vi "Trainging_OneClick.vi"() -> ()   [LabVIEW 2014]
uses:
  <vilib>/Utility/file.llb/Read From Spreadsheet File (string).vi
  <vilib>/Utility/file.llb/Read From Spreadsheet File (I64).vi
  <vilib>/Utility/file.llb/Read From Spreadsheet File (DBL).vi
  <vilib>/Utility/file.llb/Write To Spreadsheet File (DBL).vi
  <vilib>/Utility/file.llb/Write To Spreadsheet File (I64).vi
panel:
  out "error out 2":errorcluster
  out "error out":errorcluster
  out "Path_error out":errorcluster
  in  "Training_Path":path
  in  "Random_num":i32=6
  in  "Flash_Repeat":i32=20
  in  "Frame_Length":i32=20
  in  "Variables":T1={"s_verbose"=enum."On", "displayInterval"=1.0, "displayMode"=enum."On", "sampleSize"=1.0, "guess"=[[1.0]], "initState"=enum."rand", "maxFinetune"=100.0, "maxNumIteration"=100.0, "epsilon"=0.0001, "stabilization"=enum."On", "myy"=1.0, "a1"=1.0, "a2"=1.0, "finetune"=enum."off", "g"=enum."pow3", "approach"=enum."symm"}
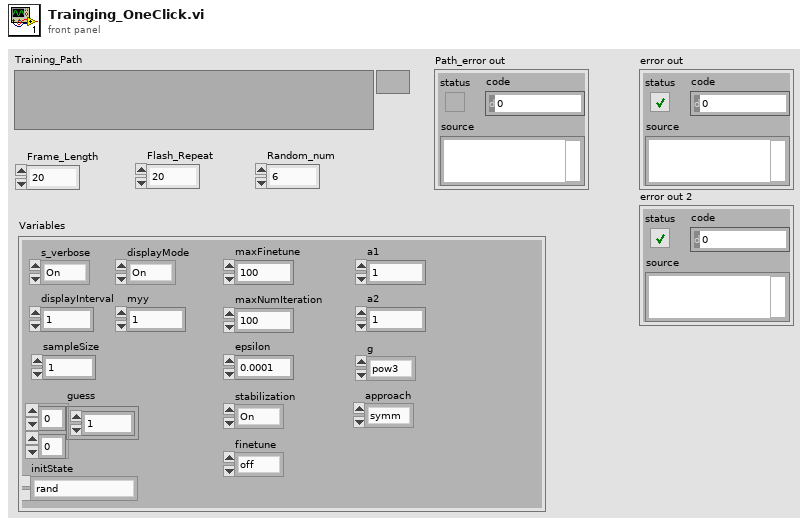
[diagram p1: front panel]
types:
  T1 = cluster{"s_verbose":enum16{"Off", "On"}, "displayInterval":dbl, "displayMode":enum16{"Off", "On"}, "sampleSize":dbl, "guess":dbl[][], "initState":enum16{"rand", "guess"}, "maxFinetune":dbl, "maxNumIteration":dbl, "epsilon":dbl, "stabilization":enum16{"Off", "On"}, "myy":dbl, "a1":dbl, "a2":dbl, "finetune":enum16{"pow3", "tanh", "gauss", "skew", "off"}, "g":enum16{"pow3", "tanh", "gauss", "skew"}, "approach":enum16{"symm", "delf"}}
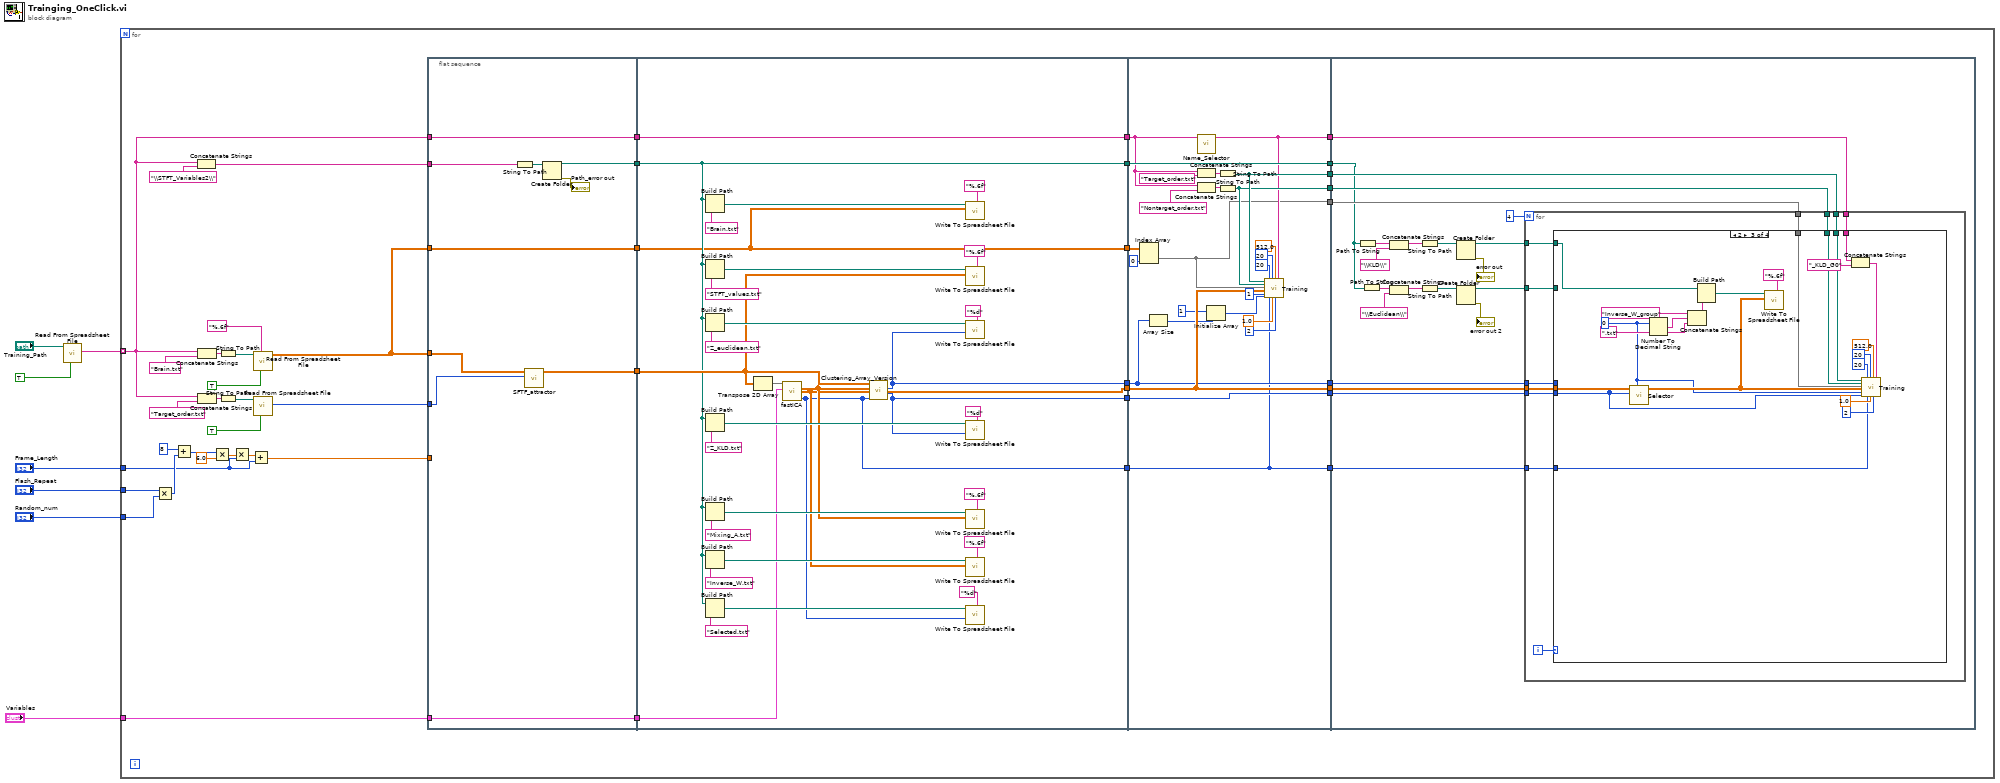
[diagram p0: block diagram]
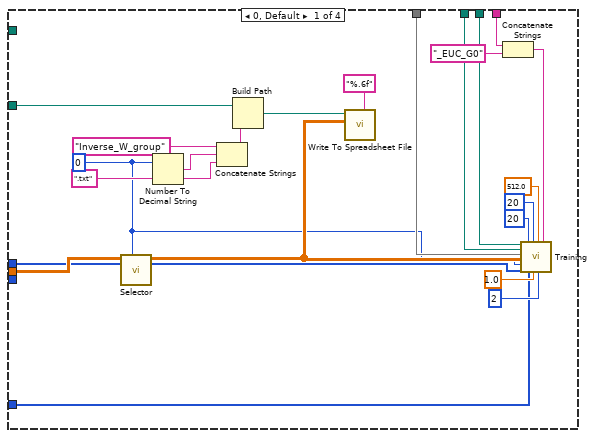
[diagram p2: hidden frame]
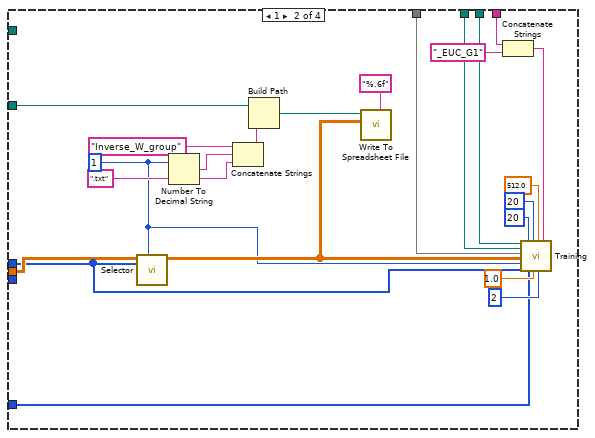
[diagram p3: hidden frame]
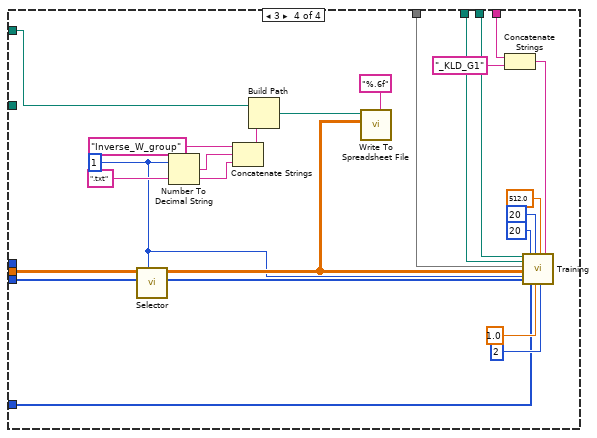
[diagram p4: hidden frame]
diagram:
  n1 = call-poly <vilib>:"Read From Spreadsheet File.vi"("transpose (no:F)"=TRUE, "file path (dialog if empty)"="Training_Path") -> ("first row"=w5:string[])  [unwired: 5 in, 4 out]
  n2 = for {
    tunnel: w5 -> [w9] mode=indexing
    tunnel: "Frame_Length" -> [w39]
    tunnel: "Flash_Repeat" -> [w38]
    tunnel: "Random_num" -> [w37]
    tunnel: "Variables" -> [w36]
    n3 = Multiply(x=w38, y=w37) -> (x*y=w48:i32)
    n4 = Add(x=8, y=w48) -> (x+y=w47:i32)
    n5 = Concatenate Strings(w9, "\\STFT_Variables2\\" ("format (%.3f)")) -> (w34:string)
    n6 = Concatenate Strings(w9, "Brain.txt" ("format (%.3f)")) -> (w41:string)
    n7 = Concatenate Strings(w9, "Target_order.txt" ("format (%.3f)")) -> (w11:string)
    n8 = Multiply(x=w47, y=6.0) -> (x*y=w45:dbl)
    n9 = String To Path(string=w41) -> (path=w40:path)
    n10 = String To Path(string=w11) -> (path=w10:path)
    n11 = Multiply(x=w45, y=w39) -> (x*y=w44:dbl)
    n12 = Add(x=w44, y=w39) -> (x+y=w43:dbl)
    n13 = call-poly <vilib>:"Read From Spreadsheet File.vi"("transpose (no:F)"=TRUE, "format (%.3f)"="%.6f", "file path (dialog if empty)"=w40) -> ("all rows"=w16:dbl[][])  [unwired: 4 in, 4 out]
    n14 = call-poly <vilib>:"Read From Spreadsheet File.vi"("transpose (no:F)"=TRUE, "file path (dialog if empty)"=w10) -> ("first row"=w8:i64[])  [unwired: 5 in, 4 out]
    n15 = flat-sequence {
      tunnel: w16 -> [w55]
      tunnel: w43 -> [_]
      tunnel: [w56] -> w53
      tunnel: w36 -> [w63]
      tunnel: [w63] -> w52
      tunnel: w34 -> [w60]
      tunnel: [w59] -> w33
      tunnel: [w58] -> w32
      tunnel: w16 -> [w58]
      tunnel: w9 -> [w57]
      tunnel: [w57] -> w23
      tunnel: w8 -> [w54]
      tunnel: w53 -> [w72]
      tunnel: w52 -> [w73]
      tunnel: w33 -> [w70]
      tunnel: w32 -> [w66]
      tunnel: [w65] -> w31
      tunnel: [w70] -> w29
      tunnel: [w69] -> w27
      tunnel: [w68] -> w25
      tunnel: w23 -> [w67]
      tunnel: [w67] -> w22
      tunnel: [w66] -> w21
      tunnel: [w64] -> w15
      tunnel: w31 -> [w107]
      tunnel: [w107] -> w30
      tunnel: w29 -> [w120]
      tunnel: [w120] -> w28
      tunnel: w27 -> [w100]
      tunnel: [w100] -> w26
      tunnel: w25 -> [w119]
      tunnel: [w119] -> w24
      tunnel: w22 -> [w106]
      tunnel: w21 -> [w109]
      tunnel: [w105] -> w20
      tunnel: [w104] -> w19
      tunnel: [w103] -> w18
      tunnel: [w102] -> w17
      tunnel: w15 -> [w96]
      tunnel: [w96] -> w14
      tunnel: w30 -> [w141]
      tunnel: w28 -> [w122]
      tunnel: w26 -> [w140]
      tunnel: w24 -> [w139]
      tunnel: w20 -> [w138]
      tunnel: w19 -> [w137]
      tunnel: w18 -> [w136]
      tunnel: w17 -> [w135]
      tunnel: w14 -> [w121]
      frame #0 {
        n16 = String To Path(string=w60) -> (path=w61:path)
        n17 = call "SFTF_attractor.vi"("Target_Flash_Order"=w54, "Brain_EEG"=w55) -> ("STFT Spectrogram {X}"=w56:dbl[][])  [unwired: 9 in]
        n18 = Create Folder(path (use dialog)=w61) -> (created path=w59:path, error out=→"Path_error out":errorcluster)  [unwired: 2 in, 1 out]
      }
      frame #1 {
        n19 = Build Path(base path=w70, name or relative path="Brain.txt") -> (appended path=w83:path)
        n20 = Build Path(base path=w70, name or relative path="STFT_values.txt") -> (appended path=w80:path)
        n21 = Build Path(base path=w70, name or relative path="Z_euclidean.txt") -> (appended path=w78:path)
        n22 = Build Path(base path=w70, name or relative path="Z_KLD.txt") -> (appended path=w74:path)
        n23 = Build Path(base path=w70, name or relative path="Mixing_A.txt") -> (appended path=w92:path)
        n24 = Build Path(base path=w70, name or relative path="Inverse_W.txt") -> (appended path=w89:path)
        n25 = Build Path(base path=w70, name or relative path="Selected.txt") -> (appended path=w87:path)
        n26 = Transpose 2D Array(2D array=w72) -> (transposed array=w95:dbl[][])
        n27 = call "fastICA.vi"("Variables"=w73, "Input Data (X)"=w95) -> ("Selected(Num)"=w64:i16[], "W"=w65:ext[][], "A"=w71:ext[][])  [unwired: 7 in]
        n28 = call "Clustering_Array_Version.vi"("Selected"=w64, "Inverse_W"=w65, "mixing_A"=w71, "STFT"=w72) -> ("Z Clustering (KDL)"=w68:i32[], "Z Clustering (EUC)"=w69:i32[])  [unwired: 4 in, 2 out]
        n29 = call-poly <vilib>:"Write To Spreadsheet File.vi"("format (%.3f)"="%.6f", "2D data"=w66, "file path (dialog if empty)"=w83) -> ()  [unwired: 5 in, 1 out]
        n30 = call-poly <vilib>:"Write To Spreadsheet File.vi"("format (%.3f)"="%.6f", "2D data"=w72, "file path (dialog if empty)"=w80) -> ()  [unwired: 5 in, 1 out]
        n31 = call-poly <vilib>:"Write To Spreadsheet File.vi"("format (%d)"="%d", "1D data"=w69, "file path (dialog if empty)"=w78) -> ()  [unwired: 5 in, 1 out]
        n32 = call-poly <vilib>:"Write To Spreadsheet File.vi"("format (%d)"="%d", "1D data"=w68, "file path (dialog if empty)"=w74) -> ()  [unwired: 5 in, 1 out]
        n33 = call-poly <vilib>:"Write To Spreadsheet File.vi"("format (%.3f)"="%.6f", "2D data"=w71, "file path (dialog if empty)"=w92) -> ()  [unwired: 5 in, 1 out]
        n34 = call-poly <vilib>:"Write To Spreadsheet File.vi"("format (%.3f)"="%.6f", "2D data"=w65, "file path (dialog if empty)"=w89) -> ()  [unwired: 5 in, 1 out]
        n35 = call-poly <vilib>:"Write To Spreadsheet File.vi"("format (%d)"="%d", "1D data"=w64, "file path (dialog if empty)"=w87) -> ()  [unwired: 5 in, 1 out]
      }
      frame #2 {
        n36 = Index Array(array=w109, index (col)=0 ("disabled index (col)")) -> (element=w102:dbl[])  [unwired: 1 in]
        n37 = Array Size(array=w100) -> (size(s)=w98:i32)
        n38 = call "Name_Selector.vi"("Path"=w106) -> ("Name"=w103:string)  [unwired: 10 in]
        n39 = Concatenate Strings(w106, "Target_order.txt" ("format (%.3f)")) -> (w111:string)
        n40 = Concatenate Strings(w106, "Nontarget_order.txt" ("format (%.3f)")) -> (w112:string)
        n41 = Initialize Array(1 ("dimension size"), w98) -> (w99:i32[])
        n42 = String To Path(string=w111) -> (path=w105:path)
        n43 = String To Path(string=w112) -> (path=w104:path)
        n44 = call "Training.vi"("Target_Flash_Order"=w105, "Nontarget_Flash_Order"=w104, "Brain_data_source"=w102, "Inverse_W"=w107, "Group_num"=1, "Selected"=w99, "Flash Repeat"=20, "전체_Selected"=w96, "Frame_Length"=20, "Channel_num"=1.0, "rate"=512.0, "Experimentation_num"=2, "피험자 이름"=w103) -> ()  [unwired: 7 in]
      }
      frame #3 {
        n45 = Path To String(path=w122) -> (string=w134:string)
        n46 = Path To String(path=w122) -> (string=w127:string)
        n47 = Concatenate Strings(w134, "\\KLD\\" ("name or relative path")) -> (w131:string)
        n48 = Concatenate Strings(w127, "\\Euclidean\\" ("name or relative path")) -> (w130:string)
        n49 = String To Path(string=w131) -> (path=w132:path)
        n50 = String To Path(string=w130) -> (path=w129:path)
        n51 = Create Folder(path (use dialog)=w132) -> (created path=w124:path, error out=→"error out":errorcluster)  [unwired: 2 in, 1 out]
        n52 = Create Folder(path (use dialog)=w129) -> (created path=w123:path, error out=→"error out 2":errorcluster)  [unwired: 2 in, 1 out]
        n53 = for {
          N: 4 -> [_]
          tunnel: w141 -> [w152]
          tunnel: w140 -> [w151]
          tunnel: w139 -> [w150]
          tunnel: w138 -> [w149]
          tunnel: w137 -> [w148]
          tunnel: w136 -> [w147]
          tunnel: w135 -> [w146]
          tunnel: w124 -> [w145]
          tunnel: w123 -> [w144]
          tunnel: w121 -> [w143]
          i -> [w153]
          n54 = case shown="2" w153 {
            tunnel: w145 -> [_ _ w216 w238]
            tunnel: w144 -> [w175 w193 _ _]
            tunnel: w152 -> [w176 w192 w215 w239]
            tunnel: w151 -> [w156 w178 _ _]
            tunnel: w150 -> [_ _ w202 w225]
            tunnel: w149 -> [w163 w182 w206 w229]
            tunnel: w148 -> [w162 w183 w207 w230]
            tunnel: w147 -> [w160 w181 w203 w228]
            tunnel: w146 -> [w158 w180 w204 w227]
            tunnel: w143 -> [w154 w177 w200 w223]
            frame 0, Default {
              w155 = 0 ("Group_Num")
              n55 = call "Selector.vi"("Group_Num"=w155, "Select"=w156, "X (input Data Array, 2D)"=w176) -> ("SubArray"=w157:dbl[][])  [unwired: 8 in]
              n56 = Number To Decimal String(number=w155) -> (decimal integer string=w171:string)  [unwired: 1 in]
              n57 = Concatenate Strings("Inverse_W_group" ("name or relative path"), w171, ".txt" ("name or relative path")) -> (w174:string)
              n58 = Build Path(base path=w175, name or relative path=w174) -> (appended path=w169:path)
              n59 = call-poly <vilib>:"Write To Spreadsheet File.vi"("format (%.3f)"="%.6f", "2D data"=w157, "file path (dialog if empty)"=w169) -> ()  [unwired: 5 in, 1 out]
              n60 = Concatenate Strings(w160, "_EUC_G0" ("string")) -> (w159:string)
              n61 = call "Training.vi"("Target_Flash_Order"=w163, "Nontarget_Flash_Order"=w162, "Brain_data_source"=w158, "Inverse_W"=w157, "Group_num"=w155, "Selected"=w156, "Flash Repeat"=20, "전체_Selected"=w154, "Frame_Length"=20, "Channel_num"=1.0, "rate"=512.0, "Experimentation_num"=2, "피험자 이름"=w159) -> ()  [unwired: 7 in]
            }
            frame 1 {
              w179 = 1 ("Group_Num")
              n62 = call "Selector.vi"("Group_Num"=w179, "Select"=w178, "X (input Data Array, 2D)"=w192) -> ("SubArray"=w184:dbl[][])  [unwired: 8 in]
              n63 = Number To Decimal String(number=w179) -> (decimal integer string=w196:string)  [unwired: 1 in]
              n64 = Concatenate Strings("Inverse_W_group" ("name or relative path"), w196, ".txt" ("name or relative path")) -> (w199:string)
              n65 = Build Path(base path=w193, name or relative path=w199) -> (appended path=w194:path)
              n66 = call-poly <vilib>:"Write To Spreadsheet File.vi"("format (%.3f)"="%.6f", "2D data"=w184, "file path (dialog if empty)"=w194) -> ()  [unwired: 5 in, 1 out]
              n67 = Concatenate Strings(w181, "_EUC_G1" ("string")) -> (w185:string)
              n68 = call "Training.vi"("Target_Flash_Order"=w182, "Nontarget_Flash_Order"=w183, "Brain_data_source"=w180, "Inverse_W"=w184, "Group_num"=w179, "Selected"=w178, "Flash Repeat"=20, "전체_Selected"=w177, "Frame_Length"=20, "Channel_num"=1.0, "rate"=512.0, "Experimentation_num"=2, "피험자 이름"=w185) -> ()  [unwired: 7 in]
            }
            frame 2 {
              w201 = 0 ("Group_Num")
              n69 = call "Selector.vi"("Group_Num"=w201, "Select"=w202, "X (input Data Array, 2D)"=w215) -> ("SubArray"=w205:dbl[][])  [unwired: 8 in]
              n70 = Number To Decimal String(number=w201) -> (decimal integer string=w219:string)  [unwired: 1 in]
              n71 = Concatenate Strings("Inverse_W_group" ("name or relative path"), w219, ".txt" ("name or relative path")) -> (w222:string)
              n72 = Build Path(base path=w216, name or relative path=w222) -> (appended path=w217:path)
              n73 = call-poly <vilib>:"Write To Spreadsheet File.vi"("format (%.3f)"="%.6f", "2D data"=w205, "file path (dialog if empty)"=w217) -> ()  [unwired: 5 in, 1 out]
              n74 = Concatenate Strings(w203, "_KLD_G0" ("string")) -> (w208:string)
              n75 = call "Training.vi"("Target_Flash_Order"=w206, "Nontarget_Flash_Order"=w207, "Brain_data_source"=w204, "Inverse_W"=w205, "Group_num"=w201, "Selected"=w202, "Flash Repeat"=20, "전체_Selected"=w200, "Frame_Length"=20, "Channel_num"=1.0, "rate"=512.0, "Experimentation_num"=2, "피험자 이름"=w208) -> ()  [unwired: 7 in]
            }
            frame 3 {
              w224 = 1 ("Group_Num")
              n76 = call "Selector.vi"("Group_Num"=w224, "Select"=w225, "X (input Data Array, 2D)"=w239) -> ("SubArray"=w226:dbl[][])  [unwired: 8 in]
              n77 = Number To Decimal String(number=w224) -> (decimal integer string=w242:string)  [unwired: 1 in]
              n78 = Concatenate Strings("Inverse_W_group" ("name or relative path"), w242, ".txt" ("name or relative path")) -> (w245:string)
              n79 = Build Path(base path=w238, name or relative path=w245) -> (appended path=w240:path)
              n80 = call-poly <vilib>:"Write To Spreadsheet File.vi"("format (%.3f)"="%.6f", "2D data"=w226, "file path (dialog if empty)"=w240) -> ()  [unwired: 5 in, 1 out]
              n81 = Concatenate Strings(w228, "_KLD_G1" ("string")) -> (w231:string)
              n82 = call "Training.vi"("Target_Flash_Order"=w229, "Nontarget_Flash_Order"=w230, "Brain_data_source"=w227, "Inverse_W"=w226, "Group_num"=w224, "Selected"=w225, "Flash Repeat"=20, "전체_Selected"=w223, "Frame_Length"=20, "Channel_num"=1.0, "rate"=512.0, "Experimentation_num"=2, "피험자 이름"=w231) -> ()  [unwired: 7 in]
            }
          }
        }
      }
    }
  }
